vi "reset AO_galvo.vi"() -> ()   [LabVIEW 2012]
doc: "SciScan 1.0 151216"
uses:
  GFG/GFGbooleanGet.vi
  <vilib>/DAQmx/create/channels.llb/DAQmx Create Channel (AO-Voltage-Basic).vi
  <vilib>/DAQmx/write.llb/DAQmx Write.vi
  <vilib>/DAQmx/write.llb/DAQmx Write (Analog 1D DBL NChan 1Samp).vi
  GFG/GFGstringGet.vi
  GFG/GFG library.lvlib
panel:
  out "error out 2":errorcluster
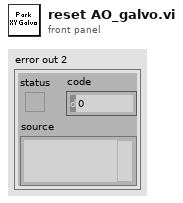
[diagram p1: front panel]
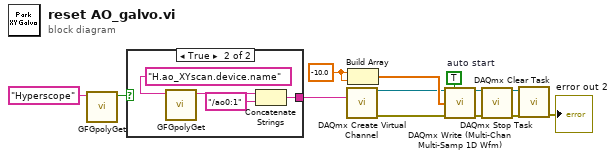
[diagram p0: block diagram]
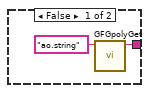
[diagram p2: hidden frame]
diagram:
  w5 = TRUE  # auto start
  w2 = -10.0 ("data")
  n1 = call-poly "GFGpolyGet.vi"("Variable Name in"="Hyperscope") -> ("Boolean Value OUT"=w12:bool)  [unwired: 9 in, 1 out]
  n2 = case shown="True" w12 {
    tunnel: [w14 w16] -> w1
    frame False {
      n3 = call-poly "GFGpolyGet.vi"("Variable Name in"="ao.string" ("name to assign")) -> ("String"=w14:string)  [unwired: 9 in, 1 out]
    }
    frame True {
      n4 = call-poly "GFGpolyGet.vi"("Variable Name in"="H.ao_XYscan.device.name" ("name to assign")) -> ("String"=w18:string)  [unwired: 9 in, 1 out]
      n5 = Concatenate Strings(w18, "/ao0:1" ("string")) -> (w16:string)
    }
  }
  n6 = call-poly <vilib>:"DAQmx Create Virtual Channel.vi"("physical channels"=w1) -> ("task out"=w4:refnum<k21>, "error out"=w6:errorcluster)  [unwired: 13 in]
  n7 = Build Array(w2, w2) -> (w11:dbl[])
  n8 = call-poly "DAQmx Write (Multi-Chan Multi-Samp 1D Wfm).vi"("task/channels in"=w4, "auto start"=w5, "data"=w11, "error in"=w6) -> ("task out"=w3:refnum<k21>, "error out"=w7:errorcluster)  [unwired: 9 in, 1 out]
  n9 = call <vilib>:"DAQmx Stop Task.vi"("task/channels in"=w3, "error in"=w7) -> ("task out"=w9:refnum<k21>, "error out"=w8:errorcluster)  [unwired: 12 in]
  n10 = call <vilib>:"DAQmx Clear Task.vi"("task in"=w9, "error in"=w8) -> ("error out"=→"error out 2":errorcluster)  [unwired: 13 in]
